vi "ma_sml_Parameter Setting for Zoom Factor (No State).vi"(7 "sml_Parameter Setting for Zoom Factor state in":T1 {"LFIR par state"."h" format="%.2f"; "CFIR par state"."h" format="%.2f"}, 10 "Reset":bool, 11 "zoom settings":T2={"zoom"=0, "aliasing protection"=enum."84 dB", "alias protect in transition band"=FALSE, "oversampling ratio"=1.0} {"oversampling ratio" format="%.2f"; "zoom" min=0}) -> (0 "comb filter order":i32, 1 "CIC Stages":i32, 2 "filter length":i32, 3 "interpolation":i32, 4 "CFIR par":cluster{"h":dbl[], "M":i32, "N":i32} {"h" format="%.2f"}, 5 "sml_Parameter Setting for Zoom Factor state out":T1 {"LFIR par state"."h" format="%.2f"; "CFIR par state"."h" format="%.2f"}, 6 "LFIR par":cluster{"h":dbl[], "M":i32, "N":i32} {"h" format="%.2f"})   [LabVIEW 2020, in "NI_MAPro.lvlib"]
uses:
  NI_MAPro.lvlib
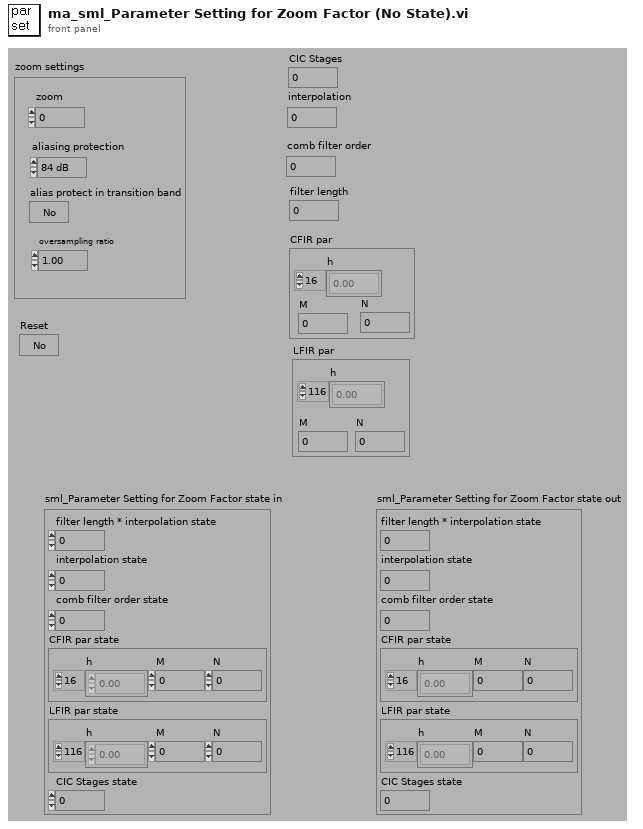
[diagram p1: front panel]
types:
  T1 = cluster{"filter length * interpolation state":i32, "interpolation state":i32, "comb filter order state":i32, "CFIR par state":cluster{"h":dbl[], "M":i32, "N":i32}, "LFIR par state":cluster{"h":dbl[], "M":i32, "N":i32}, "CIC Stages state":i32}
  T2 = cluster{"zoom":i32, "aliasing protection":enum16{"84 dB", "96 dB", "120 dB"}, "alias protect in transition band":bool, "oversampling ratio":dbl}
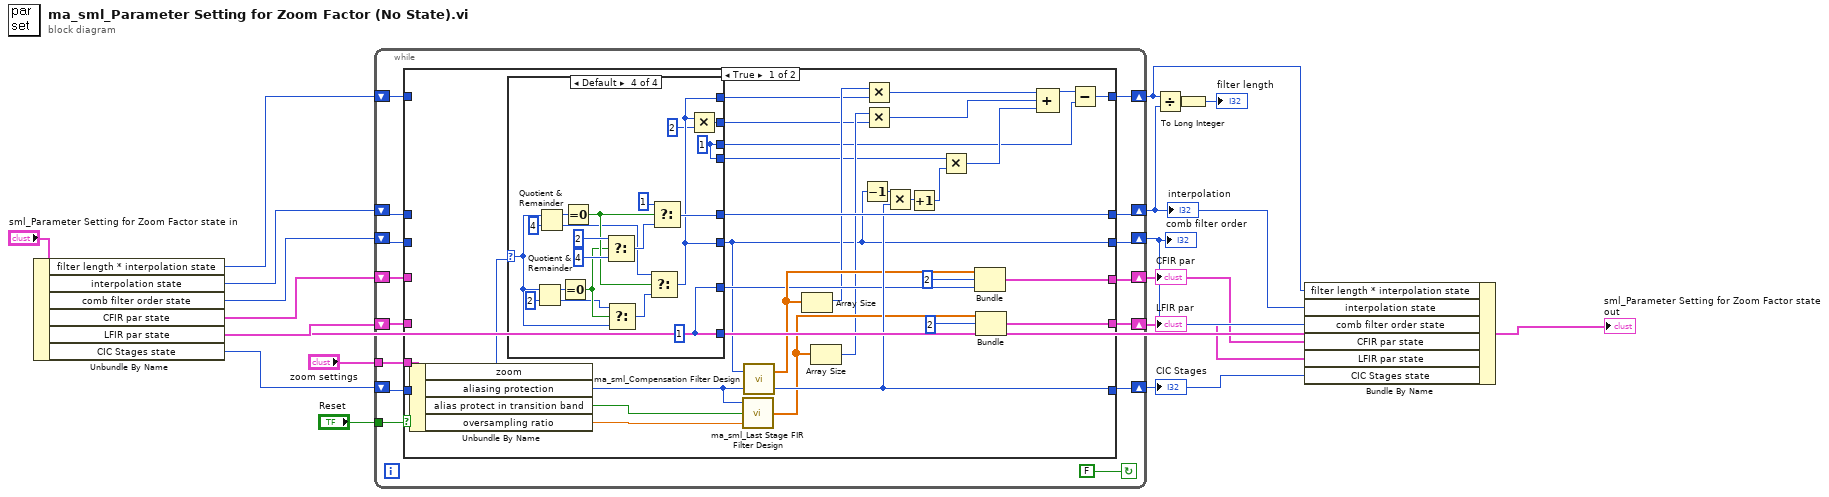
[diagram p0: block diagram]
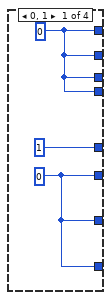
[diagram p2: hidden frame]
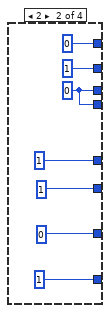
[diagram p3: hidden frame]
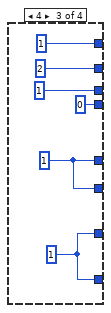
[diagram p4: hidden frame]
diagram:
  n1 = Unbundle By Name("sml_Parameter Setting for Zoom Factor state in") -> ("filter length * interpolation state"=w14:i32, "interpolation state"=w13:i32, "comb filter order state"=w12:i32, "CFIR par state"=w11:cluster{"h":dbl[], "M":i32, "N":i32}, "LFIR par state"=w10:cluster{"h":dbl[], "M":i32, "N":i32}, "CIC Stages state"=w9:i32)
  n2 = while {
    tunnel: "zoom settings" -> [w19]
    shift-left: w14 -> [w22]
    shift-right: [w23] -> w7
    shift-left: w9 -> [w24]
    shift-right: [w21] -> w1
    tunnel: "Reset" -> [w25]
    shift-left: w12 -> [w26]
    shift-right: [w29] -> w4
    shift-left: w13 -> [w27]
    shift-right: [w28] -> w5
    shift-left: w10 -> [w30]
    shift-right: [w32] -> w2
    shift-left: w11 -> [w31]
    shift-right: [w33] -> w3
    stop <- FALSE continue-if-true
    n3 = case shown="True" w25 {
      tunnel: [w61 w105] -> w33
      tunnel: [w60 w104] -> w32
      tunnel: w31 -> [_ w105]
      tunnel: w30 -> [_ w104]
      tunnel: [w35 w102] -> w29
      tunnel: [w58 w103] -> w28
      tunnel: w27 -> [_ w103]
      tunnel: w26 -> [_ w102]
      tunnel: [w57 w101] -> w21
      tunnel: w24 -> [_ w101]
      tunnel: [w40 w100] -> w23
      tunnel: w22 -> [_ w100]
      tunnel: w19 -> [w51 _]
      frame True {
        n4 = Unbundle By Name(w51) -> ("zoom"=w52:i32, "aliasing protection"=w59:enum16{"84 dB", "96 dB", "120 dB"}, "alias protect in transition band"=w55:bool, "oversampling ratio"=w54:dbl)
        n5 = case shown="Default" w52 {
          selector: w52 -> [_ _ _ w84]
          tunnel: [1 1 w78 w94] -> w58
          tunnel: [w66 1 w78 w82] -> w35
          tunnel: [w66 0 w79 w97] -> w50
          tunnel: [w66 1 w79 w97] -> w44
          tunnel: [w64 0 1 w82] -> w39
          tunnel: [w64 1 2 w83] -> w38
          tunnel: [w64 w67 1 w80] -> w37
          tunnel: [w64 w67 0 w80] -> w34
          frame 0, 1 {
            w64 = 0
            w66 = 0
          }
          frame 2 {
            w67 = 0
          }
          frame 4 {
            w79 = 1
            w78 = 1
          }
          frame Default {
            w80 = 1
            w97 = 1
            n6 = Quotient & Remainder(x=w84, y=2) -> (x-y*floor(x/y)=w96:i32, floor(x/y)=w85:i32)
            n7 = Quotient & Remainder(x=w84, y=4) -> (x-y*floor(x/y)=w98:i32, floor(x/y)=w86:i32)
            n8 = Equal To 0?(x=w96) -> (x = 0?=w87:bool)
            n9 = Equal To 0?(x=w98) -> (x = 0?=w89:bool)
            n10 = Select(t=2, s=w87, f=4) -> (s? t:f=w90:i32)
            n11 = Select(t=w85, s=w87, f=w84) -> (s? t:f=w88:i32)
            n12 = Select(t=w86, s=w89, f=w88) -> (s? t:f=w82:i32)
            n13 = Select(t=1, s=w89, f=w90) -> (s? t:f=w94:i32)
            n14 = Multiply(x=w82, y=2) -> (x*y=w83:i32)
          }
        }
        n15 = call "ma_sml_Last Stage FIR Filter Design.vi"("oversampling rate"=w54, "alias protect in final transition"=w55, "stop band attenuation"=w59) -> ("h"=w53:dbl[])
        n16 = call "ma_sml_Compensation Filter Design.vi"("stop band attenuation"=w59, "M"=w35) -> ("CIC stages"=w57:i32, "filter coefficients"=w56:dbl[])
        n17 = Array Size(array=w56) -> (size(s)=w42:i32)
        n18 = Array Size(array=w53) -> (size(s)=w43:i32)
        n19 = Decrement(x=w35) -> (x-1=w49:i32)
        n20 = Multiply(x=w42, y=w39) -> (x*y=w41:i32)
        n21 = Multiply(x=w43, y=w38) -> (x*y=w36:i32)
        n22 = Multiply(x=w49, y=w57) -> (x*y=w48:i32)
        n23 = Increment(x=w48) -> (x+1=w47:i32)
        n24 = Multiply(x=w34, y=w47) -> (x*y=w46:i32)
        n25 = Bundle("filter coefficients"=w56, 2, w50) -> (w61:cluster{"filter coefficients":dbl[], i32, i32})  [unwired: 1 out]
        n26 = Bundle("h"=w53, 2, w44) -> (w60:cluster{"h":dbl[], i32, i32})  [unwired: 1 out]
        n27 = Compound Arithmetic op=ADD(w41, w36, w46) -> (w45:i32)
        n28 = Subtract(x=w45, y=w37) -> (x-y=w40:i32)
      }
      frame False {
      }
    }
  }
  "interpolation" <- w5
  "comb filter order" <- w4
  "CFIR par" <- w3
  "LFIR par" <- w2
  "CIC Stages" <- w1
  n29 = Divide(x=w7, y=w5) -> (x/y=w17:dbl)
  n30 = To Long Integer(number=w17) -> (32bit integer=→"filter length":i32)
  n31 = Bundle By Name(cluster="sml_Parameter Setting for Zoom Factor state in", "filter length * interpolation state"=w7, "interpolation state"=w5, "comb filter order state"=w4, "CFIR par state"=w3, "LFIR par state"=w2, "CIC Stages state"=w1) -> (→"sml_Parameter Setting for Zoom Factor state out":T1)
